vi "Close Device Core.vi"(8 "error in (no error)":errorcluster, 11 "CS++Motor in":refnum<class "CS++Motor.lvclass">) -> (0 "error out":errorcluster, 3 "CS++Motor out":refnum<class "CS++Motor.lvclass">)   [LabVIEW 2015, in "CS++Motor.lvlib" / "CS++Motor.lvclass"]
doc: "Close device driver connection."
uses:
  CS++Motor.lvclass
  CSPP_Core/Actors/CS++DeviceActor/CS++DeviceActor.lvclass
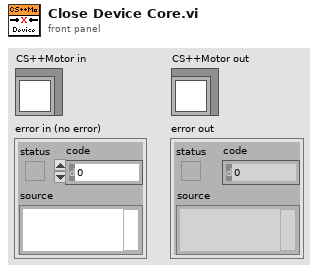
[diagram p1: front panel]
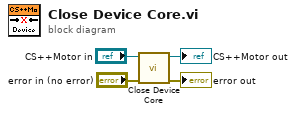
[diagram p0: block diagram]
diagram:
  n1 = call-parent "Close Device Core.vi"("error in (no error)"="error in (no error)", "CS++DeviceActor in"="CS++Motor in") -> ("error out"=→"error out":errorcluster, "CS++DeviceActor out"=→"CS++Motor out":refnum<class "CS++Motor.lvclass">)  [unwired: 8 in]
